vi "CB Get Motor Values.vi"(9 "num motors":i32=1, 11 "Motor ID":T1) -> (1 "Kt":dbl, 2 "Kv":dbl, 3 "R":dbl, 4 "motor stuff":T2)   [LabVIEW 2020]
uses:
  CB Motor ID.ctl
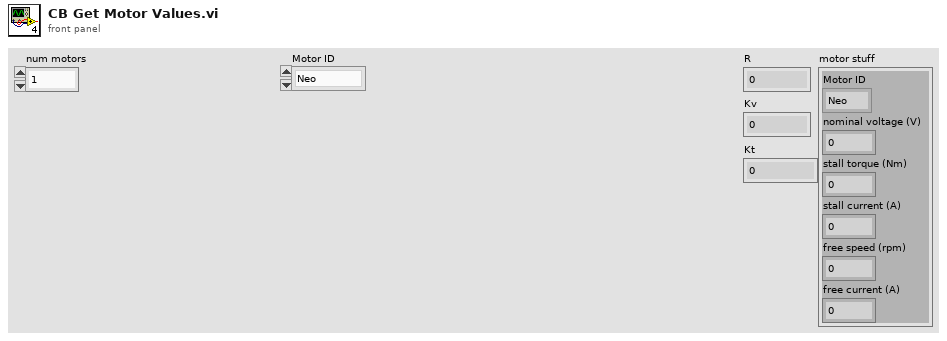
[diagram p1: front panel]
types:
  T1 = typedef "CB Motor ID.ctl" = enum16{"Neo", "Neo 550", "Falcon 500", "775pro"}
  T2 = cluster{"Motor ID":T1, "nominal voltage (V)":dbl, "stall torque (Nm)":dbl, "stall current (A)":dbl, "free speed (rpm)":dbl, "free current (A)":dbl}
  T3 = cluster{"Motor ID":T1, "nominal voltage (V)":dbl, "stall torque (Nm)":dbl, "stall current (A)":dbl, "free speed (rpm)":dbl, "free current (A)":dbl}[]
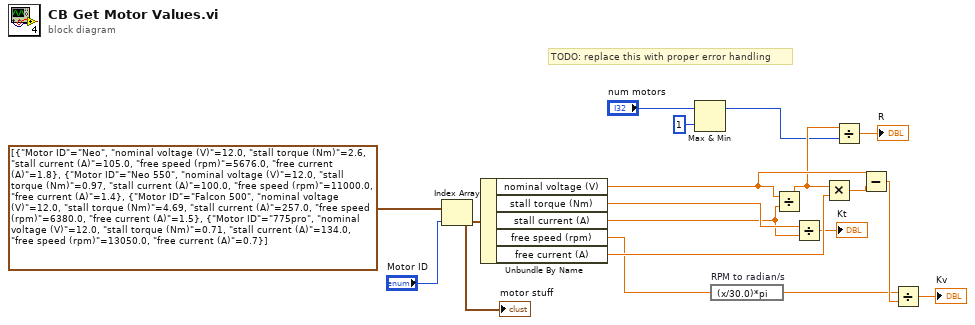
[diagram p0: block diagram]
diagram:
  # "TODO: replace this with proper error handling"
  n1 = Index Array(array=T3 [{"Motor ID"=enum."Neo", "nominal voltage (V)"=12.0, "stall torque (Nm)"=2.6, "stall current (A)"=105.0, "free speed (rpm)"=5676.0, "free current (A)"=1.8}, {"Motor ID"=enum."Neo 550", "nominal voltage (V)"=12.0, "stall torque (Nm)"=0.97, "stall current (A)"=100.0, "free speed (rpm)"=11000.0, "free current (A)"=1.4}, {"Motor ID"=enum."Falcon 500", "nominal voltage (V)"=12.0, "stall torque (Nm)"=4.69, "stall current (A)"=257.0, "free speed (rpm)"=6380.0, "free current (A)"=1.5}, {"Motor ID"=enum."775pro", "nominal voltage (V)"=12.0, "stall torque (Nm)"=0.71, "stall current (A)"=134.0, "free speed (rpm)"=13050.0, "free current (A)"=0.7}] ("appended array"), index="Motor ID") -> (element=w16:T2)
  "motor stuff" <- w16
  n2 = Unbundle By Name(w16) -> ("nominal voltage (V)"=w11:dbl, "stall torque (Nm)"=w15:dbl, "stall current (A)"=w14:dbl, "free speed (rpm)"=w7:dbl, "free current (A)"=w13:dbl)
  n3 = Max & Min(x="num motors", y=1) -> (max(x,y)=w2:i32)  [unwired: 1 out]
  n4 = expression code="(x/30.0)*pi" "RPM to radian/s"(w7) -> (w6:dbl)
  n5 = Divide(x=w11, y=w14) -> (x/y=w3:dbl)
  n6 = Divide(x=w15, y=w14) -> (x/y=→"Kt":dbl)
  n7 = Multiply(x=w3, y=w13) -> (x*y=w12:dbl)
  n8 = Divide(x=w3, y=w2) -> (x/y=→"R":dbl)
  n9 = Subtract(x=w11, y=w12) -> (x-y=w10:dbl)
  n10 = Divide(x=w6, y=w10) -> (x/y=→"Kv":dbl)
